vi "Wire Measurement Wrapper Alone.vi"(0 "vi reference":refnum<vi>, 5 "SubVI in":refnum<vi>[](array[refnum]), 7 "Terminal":refnum<vi>, 11 "error in (no error)":errorcluster) -> (15 "error out":errorcluster)   [LabVIEW 2021, in "Migrator.lvlib"]
uses:
  Migrator.lvlib
  Migrator Reusables/Migrator Reusables.lvlib
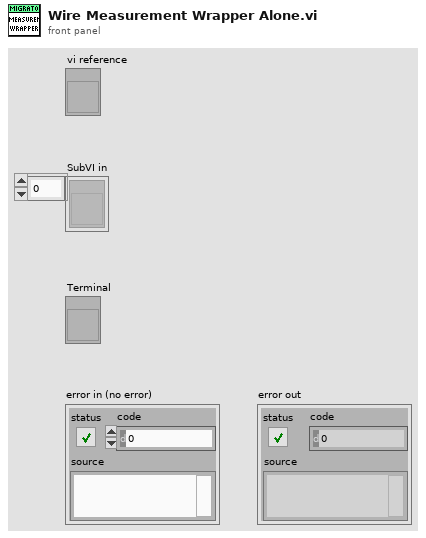
[diagram p1: front panel]
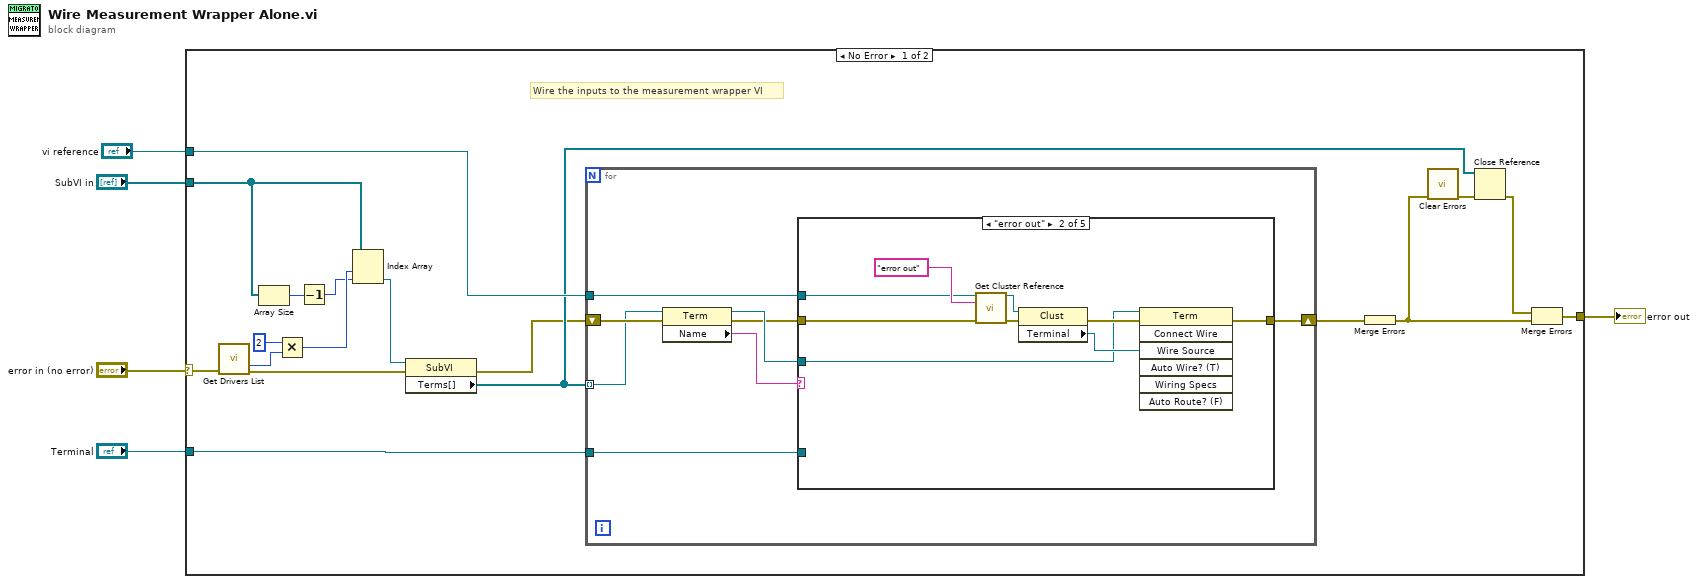
[diagram p0: block diagram]
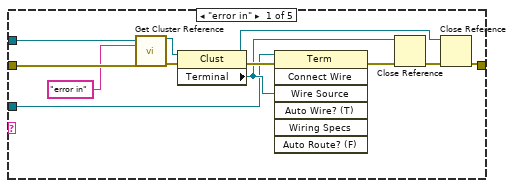
[diagram p2: hidden frame]
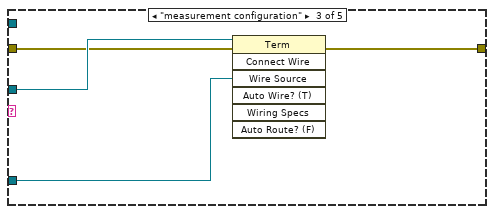
[diagram p3: hidden frame]
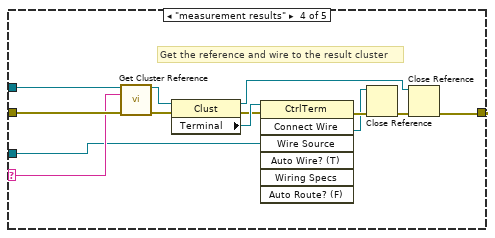
[diagram p4: hidden frame]
diagram:
  n1 = case shown="No Error" "error in (no error)" {
    selector: "error in (no error)" -> [w14 w71]
    tunnel: "vi reference" -> [w21 _]
    tunnel: [w17 w71] -> w4
    tunnel: "Terminal" -> [w15 _]
    tunnel: "SubVI in" -> [w12 _]
    frame No Error {
      # "Wire the inputs to the measurement wrapper VI"
      n2 = call "Get Drivers List.vi"("error in (no error)"=w14) -> ("Removed Duplicates Size"=w9:i32, "error out"=w13:errorcluster)  [unwired: 9 in, 4 out]
      n3 = Array Size(array=w12) -> (size(s)=w11:i32)
      n4 = Multiply(x=2, y=w9) -> (x*y=w7:i32)
      n5 = Decrement(x=w11) -> (x-1=w6:i32)
      n6 = Index Array(array=w12, index #1=w7, index #2=w6) -> (element #2=w23:refnum<vi>)  [unwired: 1 out]
      n7 = property class="SubVI"(reference=w23, error in=w13) -> (error out=w10:errorcluster, "Terms[]"=w20:refnum<vi>[])  [unwired: 1 out]
      n8 = for {
        tunnel: w20 -> [w30] mode=indexing
        tunnel: w15 -> [w29]
        tunnel: w21 -> [w28]
        shift-right: [w27] -> w22
        shift-left: w10 -> [w31]
        n9 = property class="Term"(reference=w30, error in=w31) -> (reference out=w25:refnum<vi>, error out=w24:errorcluster, "Name"=w26:string)
        n10 = case shown="\"error out\"" w26 {
          selector: w26 -> [_ _ _ w68 _]
          tunnel: w25 -> [w33 w45 w56 w64 _]
          tunnel: w29 -> [_ _ w54 _ _]
          tunnel: w24 -> [w43 w52 w55 w69 w70]
          tunnel: [w36 w51 w53 w59 w70] -> w27
          tunnel: w28 -> [w32 w44 _ w67 _]
          frame "error in" {
            n11 = call "Get Cluster Reference.vi"("VI in"=w32, "name/order"="error in", "error in (no error)"=w43) -> ("Cluster out"=w39:refnum<vi>, "error out"=w41:errorcluster)  [unwired: 11 in]
            n12 = property class="Clust"(reference=w39, error in=w41) -> (reference out=w34:refnum<vi>, error out=w38:errorcluster, "Terminal"=w35:refnum<vi>)
            n13 = invoke class="Term" method="Connect Wire"(reference=w33, error in=w38, "Wire Source"=w35) -> (error out=w42:errorcluster)  [unwired: 4 in, 6 out]
            n14 = Close Reference(reference=w35, error in (no error)=w42) -> (error out=w37:errorcluster)
            n15 = Close Reference(reference=w34, error in (no error)=w37) -> (error out=w36:errorcluster)
          }
          frame "error out" {
            n16 = call "Get Cluster Reference.vi"("VI in"=w44, "name/order"="error out", "error in (no error)"=w52) -> ("Cluster out"=w46:refnum<vi>, "error out"=w50:errorcluster)  [unwired: 11 in]
            n17 = property class="Clust"(reference=w46, error in=w50) -> (error out=w47:errorcluster, "Terminal"=w48:refnum<vi>)  [unwired: 1 out]
            n18 = invoke class="Term" method="Connect Wire"(reference=w45, error in=w47, "Wire Source"=w48) -> (error out=w51:errorcluster)  [unwired: 4 in, 6 out]
          }
          frame "measurement configuration" {
            n19 = invoke class="Term" method="Connect Wire"(reference=w56, error in=w55, "Wire Source"=w54) -> (error out=w53:errorcluster)  [unwired: 4 in, 6 out]
          }
          frame "measurement results" {
            # "Get the reference and wire to the result cluster"
            n20 = call "Get Cluster Reference.vi"("VI in"=w67, "name/order"=w68, "error in (no error)"=w69) -> ("Cluster out"=w60:refnum<vi>, "error out"=w66:errorcluster)  [unwired: 11 in]
            n21 = property class="Clust"(reference=w60, error in=w66) -> (reference out=w57:refnum<vi>, error out=w63:errorcluster, "Terminal"=w65:refnum<vi>)
            n22 = invoke class="CtrlTerm" method="Connect Wire"(reference=w65, error in=w63, "Wire Source"=w64) -> (reference out=w58:refnum<vi>, error out=w62:errorcluster)  [unwired: 4 in, 5 out]
            n23 = Close Reference(reference=w58, error in (no error)=w62) -> (error out=w61:errorcluster)
            n24 = Close Reference(reference=w57, error in (no error)=w61) -> (error out=w59:errorcluster)
          }
          frame Default {
          }
        }
      }
      n25 = Merge Errors(w22) -> (w19:errorcluster)
      n26 = call <vilib>:"Clear Errors.vi"("error in (no error)"=w19) -> ("error out"=w18:errorcluster)  [unwired: 5 in, 1 out]
      n27 = Close Reference(reference=w20, error in (no error)=w18) -> (error out=w16:errorcluster)
      n28 = Merge Errors(w16, w19) -> (w17:errorcluster)
    }
    frame Error {
    }
  }
  "error out" <- w4
